vi "setStages.vi"(8 "error in (no error)":errorcluster, 10 "Stage":string, 11 "ScriptEvent.lvclass in":refnum<class "ScriptEvent.lvclass">) -> (0 "error out":errorcluster, 3 "ScriptEvent.lvclass out":refnum<class "ScriptEvent.lvclass">)   [LabVIEW 2011, in "Tools.lvlib" / "Scripting.lvlib" / "ScriptEvent.lvclass"]
uses:
  ScriptEvent.lvclass
  ScriptEvent.lvclass/ScriptEvent.ctl
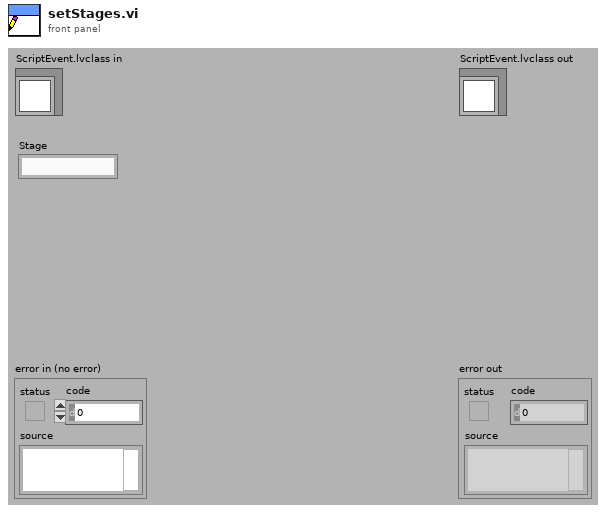
[diagram p1: front panel]
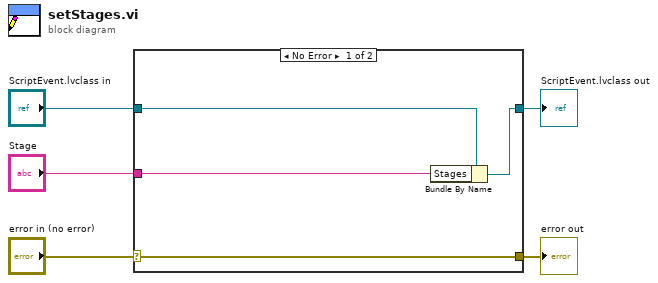
[diagram p0: block diagram]
diagram:
  n1 = case shown="No Error" "error in (no error)" {
    selector: "error in (no error)" -> [w9 w10]
    tunnel: [w9 w10] -> w4
    tunnel: [w7 w11] -> w2
    tunnel: "ScriptEvent.lvclass in" -> [w8 w11]
    tunnel: "Stage" -> [w6 _]
    frame No Error {
      n2 = Bundle By Name(cluster=w8, "Stages"=w6) -> (w7:refnum<class "ScriptEvent.lvclass">)
    }
    frame Error {
    }
  }
  "error out" <- w4
  "ScriptEvent.lvclass out" <- w2
